vi "SensorSetup.vi"   [LabVIEW 2020]
uses:
  2017 Swerve Code/Swerve Global Variables.vi
  Robot Global Data.vi
types:
  T1 = typedef "WPI_SwitchDevRef.ctl" = cluster{"DevStatus":errorcluster, "DIO Channel":T2, "CntIndex":T3, "Normally Closed":bool}
  T2 = typedef "FPGA_DIOChannel.ctl" = enum8{"DIO 0", "DIO 1", "DIO 2", "DIO 3", "DIO 4", "DIO 5", "DIO 6", "DIO 7", "DIO 8", "DIO 9", "DIO MXP 0", "DIO MXP 1", "DIO MXP 2", "DIO MXP 3", "DIO MXP 4", "DIO MXP 5", "DIO MXP 6", "DIO MXP 7", "DIO MXP 8", "DIO MXP 9", "DIO MXP 10", "DIO MXP 11", "DIO MXP 12", "DIO MXP 13", "DIO MXP 14", "DIO MXP 15", "SPI Port CS1", "SPI Port CS2", "SPI Port CS3", "SPI Port MISO", "SPI Port MOSI", "Invalid"}
  T3 = typedef "FPGA_CounterCtrSystemIndex.ctl" = enum8{"Ctr 0", "Ctr 1", "Ctr 2", "Ctr 3", "Ctr 4", "Ctr 5", "Ctr 6", "Ctr 7", "Invalid"}
  T4 = typedef "WPI_EncoderDevRef.ctl" = cluster{"DevStatus":errorcluster, "EncoderIndex":T5, "CounterIndex":T3, "DistancePerCount":dbl, "Decoding Type":T6}
  T5 = typedef "FPGA_EncoderIdx.ctl" = enum8{"Enc 0", "Enc 1", "Enc 2", "Enc 3", "Enc 4", "Enc 5", "Enc 6", "Enc 7", "Invalid"}
  T6 = typedef "WPI_EncoderType.ctl" = enum16{"1x", "2x", "4x"}
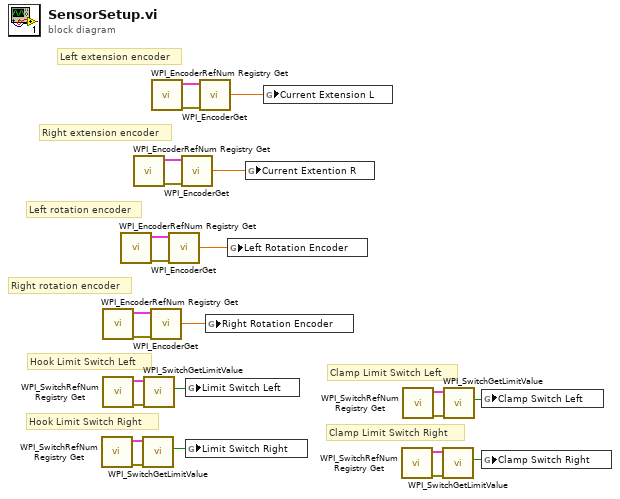
[diagram p0: block diagram]
diagram:
  # "Clamp Limit Switch Right"
  # "Clamp Limit Switch Left"
  # "Hook Limit Switch Right"
  # "Hook Limit Switch Left"
  # "Right rotation encoder"
  # "Left rotation encoder"
  # "Right extension encoder"
  # "Left extension encoder"
  n1 = call <vilib>:"WPI_SwitchRefNum Registry Get.vi"() -> ("error out"=w16:errorcluster, "SwitchDevRef"=w17:T1)  [unwired: 10 in]
  n2 = call <vilib>:"WPI_EncoderRefNum Registry Get.vi"() -> ("error out"=w10:errorcluster, "EncoderDevRef"=w11:T4)  [unwired: 10 in]
  n3 = call <vilib>:"WPI_SwitchRefNum Registry Get.vi"() -> ("error out"=w13:errorcluster, "SwitchDevRef"=w14:T1)  [unwired: 10 in]
  n4 = call <vilib>:"WPI_EncoderRefNum Registry Get.vi"() -> ("error out"=w7:errorcluster, "EncoderDevRef"=w8:T4)  [unwired: 10 in]
  n5 = call <vilib>:"WPI_EncoderRefNum Registry Get.vi"() -> ("error out"=w4:errorcluster, "EncoderDevRef"=w5:T4)  [unwired: 10 in]
  n6 = call <vilib>:"WPI_SwitchGetLimitValue.vi"("error in (no error)"=w16, "SwitchDevRef"=w17) -> ("Switch Pressed"=w18:bool)  [unwired: 7 in, 2 out]
  n7 = call <vilib>:"WPI_SwitchGetLimitValue.vi"("error in (no error)"=w13, "SwitchDevRef"=w14) -> ("Switch Pressed"=w15:bool)  [unwired: 7 in, 2 out]
  n8 = call <vilib>:"WPI_EncoderGet.vi"("error in (no error)"=w10, "EncoderDevRef"=w11) -> ("Distance"=w12:dbl)  [unwired: 4 in, 5 out]
  n9 = call <vilib>:"WPI_EncoderRefNum Registry Get.vi"() -> ("error out"=w1:errorcluster, "EncoderDevRef"=w2:T4)  [unwired: 10 in]
  n10 = call <vilib>:"WPI_EncoderGet.vi"("error in (no error)"=w7, "EncoderDevRef"=w8) -> ("Distance"=w9:dbl)  [unwired: 4 in, 5 out]
  n11 = call <vilib>:"WPI_EncoderGet.vi"("error in (no error)"=w4, "EncoderDevRef"=w5) -> ("Distance"=w6:dbl)  [unwired: 4 in, 5 out]
  n12 = global write "Robot Global Data.vi" "Limit Switch Left"(w15) -> ()
  n13 = global write "Robot Global Data.vi" "Limit Switch Right"(w18) -> ()
  n14 = call <vilib>:"WPI_EncoderGet.vi"("error in (no error)"=w1, "EncoderDevRef"=w2) -> ("Distance"=w3:dbl)  [unwired: 4 in, 5 out]
  n15 = global write "Swerve Global Variables.vi" "Right Rotation Encoder"(w12) -> ()
  n16 = global write "Swerve Global Variables.vi" "Left Rotation Encoder"(w9) -> ()
  n17 = global write "Swerve Global Variables.vi" "Current Extention R"(w6) -> ()
  n18 = global write "Swerve Global Variables.vi" "Current Extension L"(w3) -> ()
  n19 = call <vilib>:"WPI_SwitchRefNum Registry Get.vi"() -> ("error out"=w22:errorcluster, "SwitchDevRef"=w23:T1)  [unwired: 10 in]
  n20 = call <vilib>:"WPI_SwitchRefNum Registry Get.vi"() -> ("error out"=w19:errorcluster, "SwitchDevRef"=w20:T1)  [unwired: 10 in]
  n21 = call <vilib>:"WPI_SwitchGetLimitValue.vi"("error in (no error)"=w22, "SwitchDevRef"=w23) -> ("Switch Pressed"=w24:bool)  [unwired: 7 in, 2 out]
  n22 = call <vilib>:"WPI_SwitchGetLimitValue.vi"("error in (no error)"=w19, "SwitchDevRef"=w20) -> ("Switch Pressed"=w21:bool)  [unwired: 7 in, 2 out]
  n23 = global write "Robot Global Data.vi" "Clamp Switch Left"(w21) -> ()
  n24 = global write "Robot Global Data.vi" "Clamp Switch Right"(w24) -> ()
